vi "WPI_CameraUpdate Camera Status.vi"(3 "CameraDevRef In":T1, 4 "Enable Vision":bool) -> (0 "CameraDevRef Out":T1)   [LabVIEW 2017]
doc: "This VI is used to enable or disable a camera on the robot. Internally, it caches the state of the camera, so it is safe and inexpensive to call this repeatedly in your acquisition loop."
uses:
  <vilib>/Rock Robotics/WPI/Camera/WPI_CameraDevRef.ctl
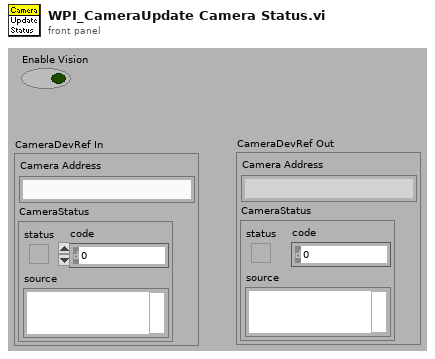
[diagram p1: front panel]
types:
  T1 = typedef "WPI_CameraDevRef.ctl" = cluster{"Camera Address":string, "CameraStatus":errorcluster}
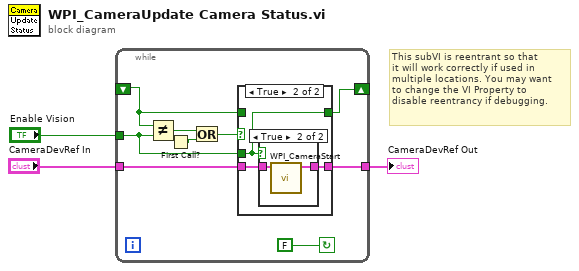
[diagram p0: block diagram]
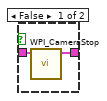
[diagram p3: hidden frame]
diagram:
  # "This subVI is reentrant so that\nit will work correctly if used in\nmultiple locations. You may want\nto change the VI Property to\ndisable reentrancy if debugging."
  n1 = while {
    tunnel: "Enable Vision" -> [w12]
    tunnel: "CameraDevRef In" -> [w11]
    tunnel: [w10] -> w1
    shift-right: [w8] -> _
    shift-left: _ -> [w9]
    stop <- FALSE continue-if-true
    n2 = Not Equal?(x=w9, y=w12) -> (x != y?=w6:bool)
    n3 = First Call?() -> (First Call?: T/F=w4:bool)
    n4 = Or(x=w6, y=w4) -> (x .or. y?=w5:bool)
    n5 = case shown="True" w5 {
      tunnel: w11 -> [w14 w17]
      tunnel: [w14 w16] -> w10
      tunnel: [w13 w15] -> w8
      tunnel: w9 -> [w13 _]
      tunnel: w12 -> [_ w15]
      frame False {
      }
      frame True {
        n6 = case shown="True" w15 {
          tunnel: w17 -> [w19 w20]
          tunnel: [w18 w21] -> w16
          frame False {
            n7 = call <vilib>:"WPI_CameraStop.vi"("CameraDevRef"=w19) -> ("CameraDevRef"=w18:T1)  [unwired: 1 in, 9 out]
          }
          frame True {
            n8 = call <vilib>:"WPI_CameraStart.vi"("CameraDevRef"=w20) -> ("CameraDevRef"=w21:T1)  [unwired: 1 in, 9 out]
          }
        }
      }
    }
  }
  "CameraDevRef Out" <- w1
